vi "Configure GPIO Pin.vi"(0 "VISA resource name":refnum<visa-resource-name>, 1 "GPIO Pin Trigger Type (0: Edge)":i32(ring) items=["Edge", "Level"], 2 "GPIO Pin Output Data (0)":i32, 5 "Pin Number (1)":i32=1, 7 "GPIO Pin I/O Function (0: Digital Input)":i32(ring) items=["Digital Input", "Digital I/O", "Trigger Input", "Trigger Output"], 9 "GPIO Pin Polarity (0: Negative)":i32(ring) items=["Negative", "Positive"], 11 "error in (no error)":errorcluster, 12 "GPIO Pin Trigger Timing (2: Both)":i32(ring)=2 items=["Before", "After", "Both"], 13 "GPIO Pin Trigger Pulse Width (0.0001 s)":dbl=0.0001) -> (4 "VISA resource name out":refnum<visa-resource-name>, 15 "error out":errorcluster)   [LabVIEW 2012, in "Keysight B2980 Series.lvlib"]
doc: "Configure GPIO(General Purpose I/O) Pin, which is an I/O port of the Digital I/O D-sub connector on the rear panel.\n\n<b>Note(s):</b>\nThis VI is only applicable for model B2985A and B2987A."
uses:
  Keysight B2980 Series.lvlib
panel:
  # "GPIO Pin Trigger Settings"
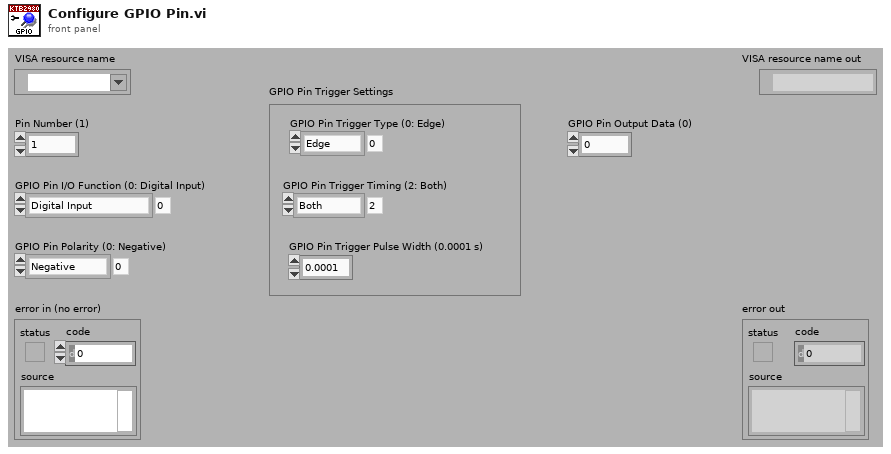
[diagram p1: front panel]
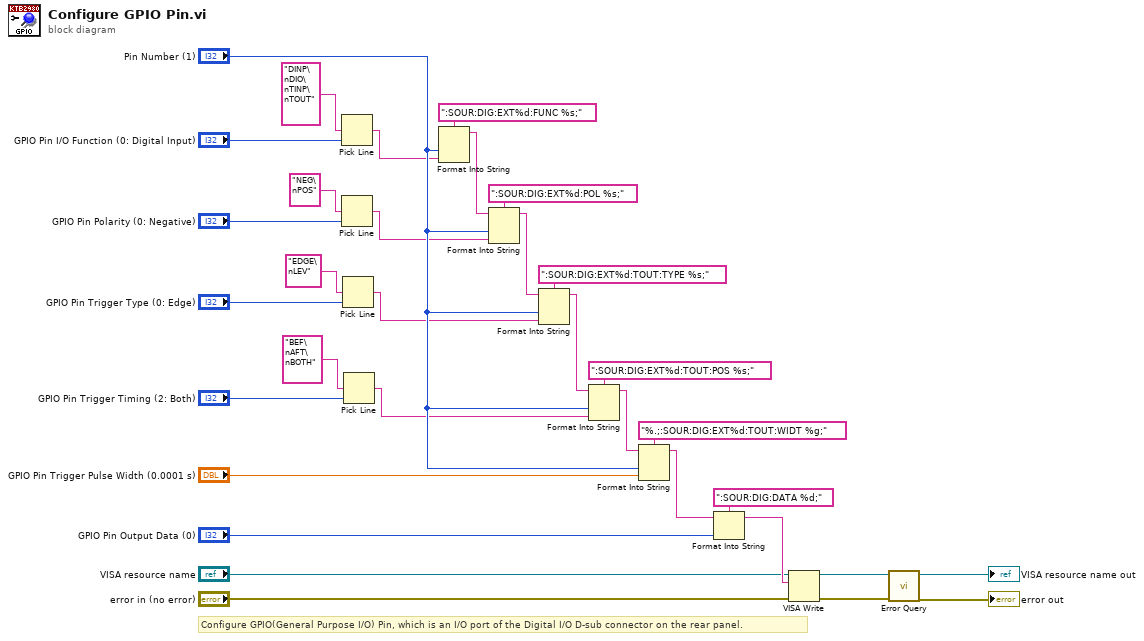
[diagram p0: block diagram]
diagram:
  # "Configure GPIO(General Purpose I/O) Pin, which is an I/O port of the Digital I/O D-sub connector on the rear panel."
  n1 = Pick Line(multi-line string="DINP\nDIO\nTINP\nTOUT", line index="GPIO Pin I/O Function (0: Digital Input)") -> (output string=w29:string)  [unwired: 1 out]
  n2 = Pick Line(multi-line string="NEG\nPOS", line index="GPIO Pin Polarity (0: Negative)") -> (output string=w24:string)  [unwired: 1 out]
  n3 = Pick Line(multi-line string="EDGE\nLEV", line index="GPIO Pin Trigger Type (0: Edge)") -> (output string=w19:string)  [unwired: 1 out]
  n4 = Pick Line(multi-line string="BEF\nAFT\nBOTH", line index="GPIO Pin Trigger Timing (2: Both)") -> (output string=w14:string)  [unwired: 1 out]
  n5 = Format Into String(format string=":SOUR:DIG:EXT%d:FUNC %s;", "Pin Number (1)", w29) -> (resulting string=w26:string)  [unwired: 2 in, 1 out]
  n6 = Format Into String(format string=":SOUR:DIG:EXT%d:POL %s;", initial string=w26, "Pin Number (1)", w24) -> (resulting string=w21:string)  [unwired: 1 in, 1 out]
  n7 = Format Into String(format string=":SOUR:DIG:EXT%d:TOUT:TYPE %s;", initial string=w21, "Pin Number (1)", w19) -> (resulting string=w16:string)  [unwired: 1 in, 1 out]
  n8 = Format Into String(format string=":SOUR:DIG:EXT%d:TOUT:POS %s;", initial string=w16, "Pin Number (1)", w14) -> (resulting string=w13:string)  [unwired: 1 in, 1 out]
  n9 = Format Into String(format string="%.;:SOUR:DIG:EXT%d:TOUT:WIDT %g;", initial string=w13, "Pin Number (1)", "GPIO Pin Trigger Pulse Width (0.0001 s)") -> (resulting string=w10:string)  [unwired: 1 in, 1 out]
  n10 = Format Into String(format string=":SOUR:DIG:DATA %d;", initial string=w10, "GPIO Pin Output Data (0)") -> (resulting string=w7:string)  [unwired: 1 in, 1 out]
  n11 = VISA Write(VISA resource name="VISA resource name", write buffer=w7, error in (no error)="error in (no error)") -> (VISA resource name out=w4:refnum<visa-resource-name>, error out=w3:errorcluster)  [unwired: 1 out]
  n12 = call "Error Query.vi"("error in (no error)"=w3, "VISA resource name"=w4) -> ("error out"=→"error out":errorcluster, "VISA resource name out"=→"VISA resource name out":refnum<visa-resource-name>)  [unwired: 8 out]
